vi "Estimate Time.vi"(8 "error in (no error)":errorcluster, 11 "Scan Driver in":refnum<class "Scan Driver.lvclass">) -> (0 "error out":errorcluster, 1 "Seconds":dbl[unit], 2 "Time Estimate":string, 3 "Scan Driver out":refnum<class "Scan Driver.lvclass">)   [LabVIEW 2009, in "Scan Driver.lvclass"]
doc: "Estimate the time needed to complete this Scan Driver instance, using data from member Scanner and Reader."
uses:
  Scan Driver.lvclass
  Scan Driver.lvclass/Scan Driver.ctl
  Readers/Reader/Reader.lvclass
  Scanners/Scanner/Scanner.lvclass
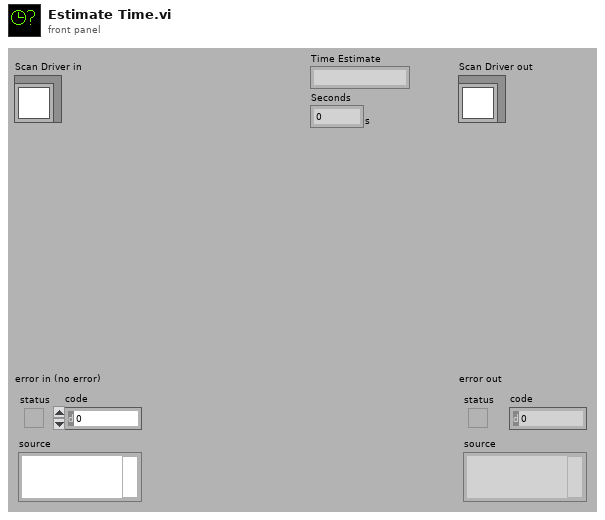
[diagram p1: front panel]
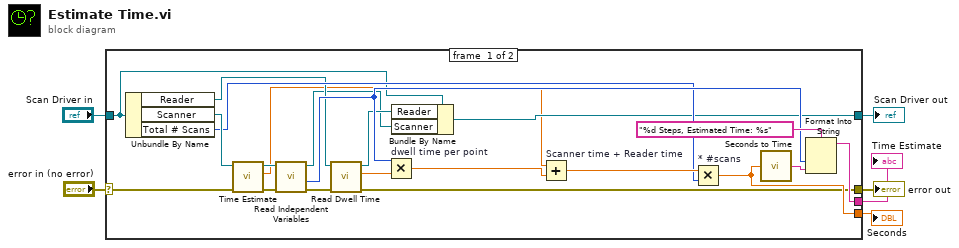
[diagram p0: block diagram]
diagram:
  n1 = case shown="No Error" "error in (no error)" {
    selector: "error in (no error)" -> [w9 w29]
    tunnel: [w22 _] -> w2
    tunnel: [w21 _] -> w1
    tunnel: [w13 w28] -> w5
    tunnel: [w7 w29] -> w6
    tunnel: "Scan Driver in" -> [w12 w28]
    frame #0 {
      n2 = Unbundle By Name(w12) -> ("Reader"=w17:refnum<class "Reader.lvclass">, "Scanner"=w20:refnum<class "Scanner.lvclass">, "Total # Scans"=w18:u32)
      n3 = call-dynamic "Time Estimate.vi"("error in (no error)"=w9, "Scanner.lvclass"=w20) -> ("error out"=w11:errorcluster, "time"=w10:dbl[unit], "Scanner.lvclass out"=w19:refnum<class "Scanner.lvclass">)  [unwired: 2 in, 5 out]
      n4 = call-dynamic "Read Independent Variables.vi"("error in (no error)"=w11, "Scanner.lvclass in"=w19) -> ("error out"=w8:errorcluster, "size"=w23:i32, "Scanner.lvclass out"=w14:refnum<class "Scanner.lvclass">)  [unwired: 7 out]
      n5 = call-dynamic "Read Dwell Time.vi"("error in (no error)"=w8, "Reader.lvclass in"=w17) -> ("error out"=w7:errorcluster, "Dwell Time"=w16:dbl[unit], "Reader.lvclass out"=w15:refnum<class "Reader.lvclass">)  [unwired: 7 out]
      n6 = Multiply "dwell time per point"(x=w23, y=w16) -> (x*y=w27:dbl[unit])
      n7 = Bundle By Name(cluster=w12, "Reader"=w15, "Scanner"=w14) -> (w13:refnum<class "Scan Driver.lvclass">)
      n8 = Add "Scanner time + Reader time"(x=w10, y=w27) -> (x+y=w26:dbl[unit])
      n9 = Multiply "* #scans"(x=w26, y=w18) -> (x*y=w21:dbl[unit])
      n10 = call "Seconds to Time.vi"("Seconds"=w21) -> ("Time"=w24:string)
      n11 = Format Into String(format string="%d Steps, Estimated Time: %s", w23, w24) -> (resulting string=w22:string)  [unwired: 2 in, 1 out]
    }
    frame #1 {
    }
  }
  "error out" <- w6
  "Scan Driver out" <- w5
  "Time Estimate" <- w2
  "Seconds" <- w1
